vi "RT.vi"() -> ()   [LabVIEW 2018]
uses:
  <vilib>/FPGAPlugInAG/sbRIO-9607/niLvFpga_Open_sbRIO-9607.vi
  <vilib>/rvi/interface/common/dynamic/niFpgaDynamicAddResources.vi
  <vilib>/Utility/error.llb/Error Cluster From Error Code.vi
  <vilib>/rvi/errors/niLvFpgaAdjustHostInterfaceError.vi
  <vilib>/FPGAPlugInAG/Dynamic/niLvFpga_Close_Dynamic.vi
  <vilib>/rvi/interface/nirviOpenFPGA/nirviOpenFPGA.xnode
  FPGA Bitfiles/SPIFast_FPGATarget_FPGA_QLB7yT0DmFg.lvbitx
  FPGA.vi
  <vilib>/rvi/interface/nirviReadWriteControl/nirviReadWriteControl.xnode
  <vilib>/rvi/interface/nirviCloseFPGA/nirviCloseFPGA.xnode
  NiFpgaLv.dll
  <vilib>/rvi/interface/Simulation/niFpgaSimulationCallBeginRW.vi
panel:
  in  "SP 4":u8
  in  "SP 3":u8
  in  "SP 2":u8
  in  "SP":u8
  out "Byte 3":u8
  out "Byte 2":u8
  out "Byte 1":u8
  out "Byte 0":u8
  in  "Stop Button":bool
  in  "Pause":u8=20
  in  "Clock":u8=180
  in  "SPI":bool
  out "Error Out":errorcluster
  in  "Error In":errorcluster
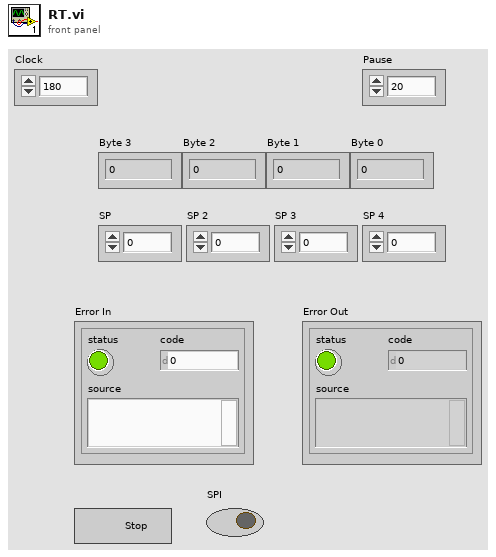
[diagram p1: front panel]
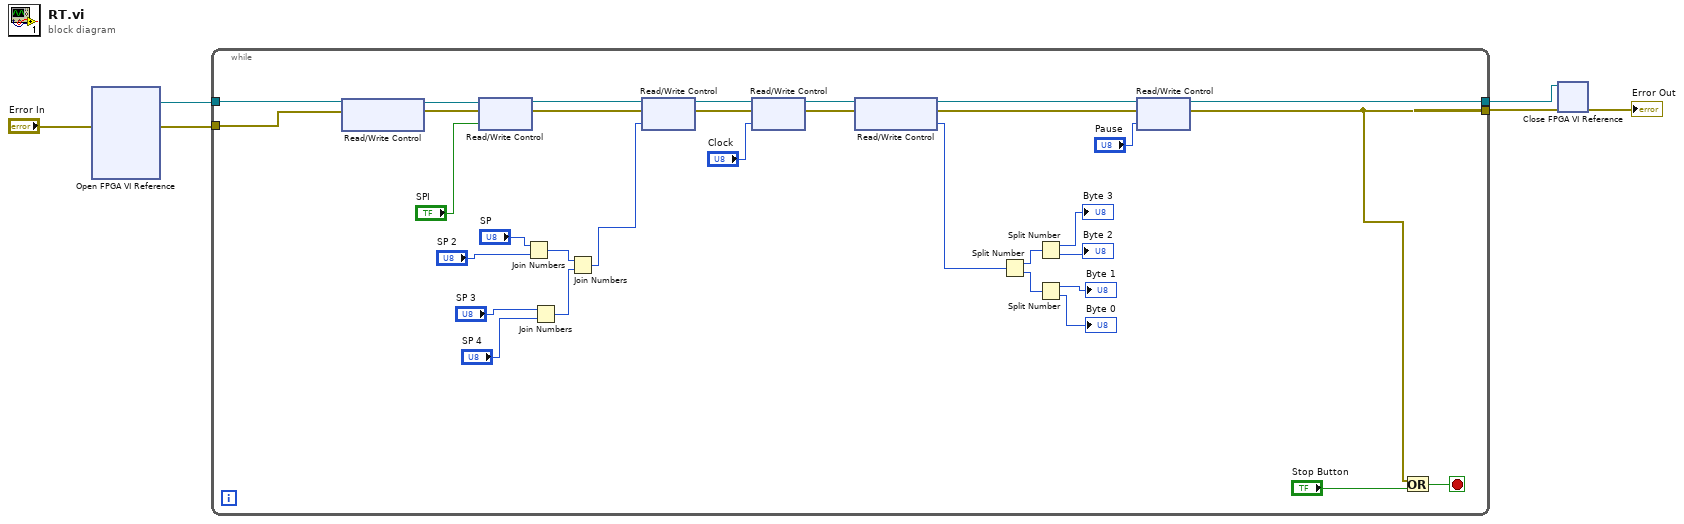
[diagram p0: block diagram]
diagram:
  n1 = xnode "Open FPGA VI Reference"("error in"="Error In") -> ("FPGA VI Reference Out"=w6:refnum<k20>, "error out"=w5:errorcluster)  [unwired: 1 in]
  n2 = while {
    tunnel: w6 -> [w33]
    tunnel: w5 -> [w28]
    tunnel: [w21] -> w2
    tunnel: [w22] -> w1
    stop <- w24 stop-if-true
    n3 = xnode "Read/Write Control"("FPGA VI Reference In"=w33, "error in"=w28) -> ("FPGA VI Reference Out"=w32:refnum<k20>, "error out"=w29:errorcluster)  [unwired: 1 out]
    n4 = xnode "Read/Write Control"("FPGA VI Reference In"=w32, "error in"=w29, "Write"="SPI") -> ("FPGA VI Reference Out"=w31:refnum<k20>, "error out"=w30:errorcluster)
    n5 = Join Numbers(hi="SP", lo="SP 2") -> ((hi.lo)=w14:u16)
    n6 = Join Numbers(hi="SP 3", lo="SP 4") -> ((hi.lo)=w13:u16)
    n7 = Join Numbers(hi=w14, lo=w13) -> ((hi.lo)=w8:u32)
    n8 = xnode "Read/Write Control"("FPGA VI Reference In"=w31, "error in"=w30, "Data"=w8) -> ("FPGA VI Reference Out"=w36:refnum<k20>, "error out"=w37:errorcluster)
    n9 = xnode "Read/Write Control"("FPGA VI Reference In"=w36, "error in"=w37, "Delay"="Clock") -> ("FPGA VI Reference Out"=w38:refnum<k20>, "error out"=w39:errorcluster)
    n10 = xnode "Read/Write Control"("FPGA VI Reference In"=w38, "error in"=w39) -> ("FPGA VI Reference Out"=w26:refnum<k20>, "error out"=w27:errorcluster, "PIC Monitor"=w7:u32)
    n11 = Split Number(x=w7) -> (hi(x)=w19:u16, lo(x)=w20:u16)
    n12 = Split Number(x=w19) -> (hi(x)=→"Byte 3":u8, lo(x)=→"Byte 2":u8)
    n13 = Split Number(x=w20) -> (hi(x)=→"Byte 1":u8, lo(x)=→"Byte 0":u8)
    n14 = xnode "Read/Write Control"("FPGA VI Reference In"=w26, "error in"=w27, "Pause"="Pause") -> ("FPGA VI Reference Out"=w22:refnum<k20>, "error out"=w21:errorcluster)
    n15 = Or(x=w21, y="Stop Button") -> (x .or. y?=w24:bool)
  }
  n16 = xnode "Close FPGA VI Reference"("FPGA VI Reference In"=w1, "error in"=w2) -> ("error out"=→"Error Out":errorcluster)
